vi "draw_overlay_in_pixel_coordinates.vi"(0 "Image in":refnum<class "Image.lvclass">, 1 "coordinates":cluster{"X":i32, "Y":i32}[](array[cluster]), 3 "overlay group":string, 5 "x coordinates":i32[](array[numeric]), 9 "y coordinates":i32[](array[numeric]), 11 "error in (no error)":errorcluster, 12 "colour":u32(colorbox)=16711680, 13 "connect points? (T)":bool=TRUE, 14 "clear previous overlay of this group? (T)":bool=TRUE) -> (4 "Image out":refnum<class "Image.lvclass">, 15 "error out":errorcluster)   [LabVIEW 2010, in "Image.lvclass"]
uses:
  Image.lvclass
  ErrorController/ErrorController/class_data.vi
  ErrorController/ErrorController/ErrorController.lvclass
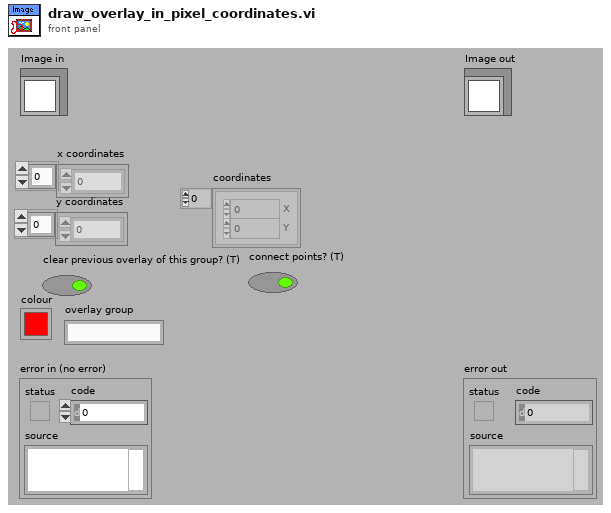
[diagram p1: front panel]
types:
  T1 = typedef "IMAQ Image.ctl" = refnum<image>
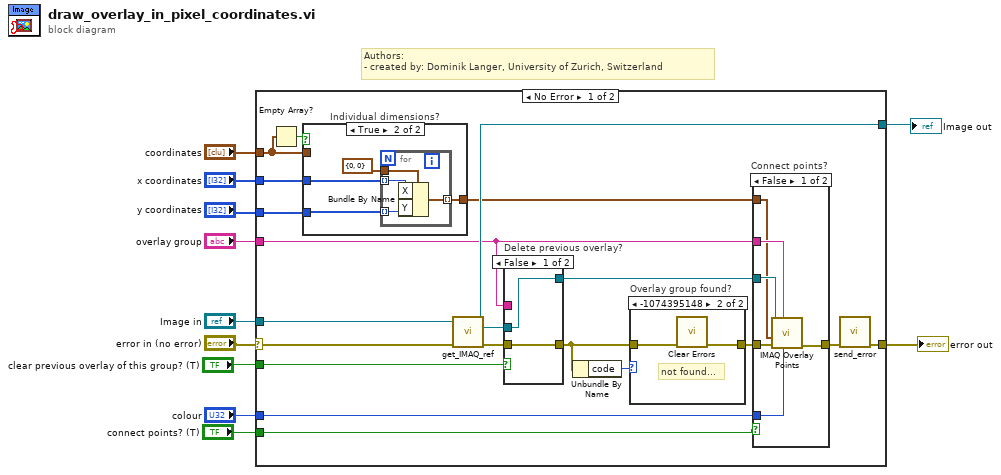
[diagram p0: block diagram]
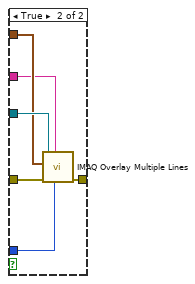
[diagram p2: hidden frame]
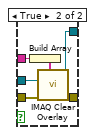
[diagram p3: hidden frame]
diagram:
  # "Authors: \n- created by: Dominik Langer, University of Zurich, Switzerland"
  n1 = case shown="No Error" "error in (no error)" {
    selector: "error in (no error)" -> [w29 w65]
    tunnel: [w13 w65] -> w8
    tunnel: [w27 w64] -> w7
    tunnel: "Image in" -> [w28 w64]
    tunnel: "x coordinates" -> [w31 _]
    tunnel: "y coordinates" -> [w30 _]
    tunnel: "colour" -> [w26 _]
    tunnel: "coordinates" -> [w17 _]
    tunnel: "overlay group" -> [w16 _]
    tunnel: "clear previous overlay of this group? (T)" -> [w15 _]
    tunnel: "connect points? (T)" -> [w14 _]
    frame No Error {
      n2 = Empty Array?(array=w17) -> (empty?=w18:bool)
      n3 = case "Individual dimensions?" shown="True" w18 {
        tunnel: w31 -> [_ w54]
        tunnel: w30 -> [_ w53]
        tunnel: [w52 w55] -> w19
        tunnel: w17 -> [w52 _]
        frame False {
        }
        frame True {
          n4 = for {
            tunnel: [w60] -> w55 mode=indexing
            tunnel: cluster{"X":i32, "Y":i32} {"X"=0, "Y"=0} ("Point Coordinates") -> [w59]
            tunnel: w54 -> [w58] mode=indexing
            tunnel: w53 -> [w57] mode=indexing
            n5 = Bundle By Name(cluster=w59, "X"=w58, "Y"=w57) -> (w60:cluster{"X":i32, "Y":i32})
          }
        }
      }
      n6 = call-dynamic "get_IMAQ_ref.vi"("error in (no error)"=w29, "Image.lvclass in"=w28) -> ("error out"=w25:errorcluster, "Image"=w24:T1, "Image.lvclass out"=w27:refnum<class "Image.lvclass">)  [unwired: 5 in, 2 out]
      n7 = case "Delete previous overlay?" shown="False" w15 {
        tunnel: w25 -> [w45 w51]
        tunnel: w24 -> [w44 w50]
        tunnel: [w45 w48] -> w23
        tunnel: [w44 w47] -> w20
        tunnel: w16 -> [_ w46]
        frame False {
        }
        frame True {
          n8 = Build Array(w46) -> (w49:string[])
          n9 = call "IMAQ Clear Overlay"("Groups"=w49, "error in (no error)"=w51, "Image"=w50) -> ("error out"=w48:errorcluster, "Image Out"=w47:T1)  [unwired: 7 in]
        }
      }
      n10 = Unbundle By Name(w23) -> ("code"=w21:i32)
      n11 = case "Overlay group found?" shown="-1074395148" w21 {
        tunnel: w23 -> [w61 w63]
        tunnel: [w61 w62] -> w22
        frame Default {
          # "either found or some other error..."
        }
        frame -1074395148 {
          # "not found..."
          n12 = call <vilib>:"Clear Errors.vi"("error in (no error)"=w63) -> ("error out"=w62:errorcluster)  [unwired: 6 in]
        }
      }
      n13 = case "Connect points?" shown="False" w14 {
        tunnel: [w36 w43] -> w12
        tunnel: w26 -> [w35 w42]
        tunnel: w22 -> [w37 w41]
        tunnel: w20 -> [w33 w40]
        tunnel: w19 -> [w32 w39]
        tunnel: w16 -> [w34 w38]
        frame False {
          n14 = call "IMAQ Overlay Points"("Color"=w35, "Group"=w34, "error in (no error)"=w37, "Array of Points"=w32, "Image"=w33) -> ("error out"=w36:errorcluster)  [unwired: 5 in, 1 out]
        }
        frame True {
          n15 = call "IMAQ Overlay Multiple Lines"("Color"=w42, "Group"=w38, "error in (no error)"=w41, "Line End Points"=w39, "Image"=w40) -> ("error out"=w43:errorcluster)  [unwired: 5 in, 1 out]
        }
      }
      n16 = call "send_error.vi"("error in (no error)"=w12) -> ("error out"=w13:errorcluster)  [unwired: 10 in]
    }
    frame Error {
    }
  }
  "error out" <- w8
  "Image out" <- w7
